vi "DAC Memory Fill [DFIL].vi"(7 "Micropulse # In":i32, 8 "error in (no error)":errorcluster, 9 "Gain (dB)":dbl min=-6.0 max=70.0 step=0.25 format="%.2fdB", 10 "End Addr":i32, 11 "Start Addr":i32) -> (0 "error out":errorcluster, 5 "Micropulse # Out":i32)   [LabVIEW 2026, in "MicroPulse_Driver.lvlib"]
doc: "Fills all addresses from address 1 to address 2 with the specified value. The addresses are within the range 0 to 65530 for standard DAC and the range 70000 to 70511 for water path DAC used in FMC echo gate mode. This command is useful for gain gating specific signals at specific ranges.\n\nParameters:\n<Addr 1> : Start address from which the specified value is to fill. Integer number between 0 and 65530 or 70000 and 70511\n\n<Addr 2> : End address to which the specified value is filled Integer number between 0 and 65530 or 70000 and 70511\n\n<Value> : Integer number representing a gain increase in 0.25 dB steps: 0 - 280 (0 - 70dB).\nThe address and value may be entered in decimal or hexadecimal Formats.\n\nExample:\nDFIL 100 200 20 : Fill from absolute address 100 to absolute address 200 with gain value 5dB.\n\nDFIL 20H C0H 120 : Fill from HEX address 20 to HEX address C0 with gain value 30.0dB"
uses:
  MicroPulse_Driver.lvlib
  Private/MP-Registry Action-Enum.ctl
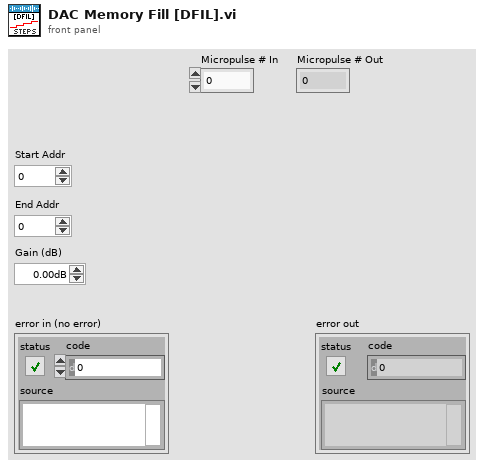
[diagram p1: front panel]
types:
  T1 = typedef "MicroPulse_Driver.lvlib/MP-Registry Action-Enum.ctl" = enum16{"Read", "Add Test", "Add Command", "Add Gate Command", "Add Encoder Command", "Clear Command  List", "Set Registry", "Set System Details", "Set DOF", "Set Velocity", "Disable Asynch Reads", "Enable Asynch Reads", "Add Connection", "Disconnect", "Shutdown"}
  T2 = typedef "MicroPulse_Driver.lvlib/TCP config.ctl" = cluster{"Connection ID":refnum<k5>, "IP address":string, "host port":u16, "OC timeout":i32, "Read timeout":i32, "Write timeout":i32}
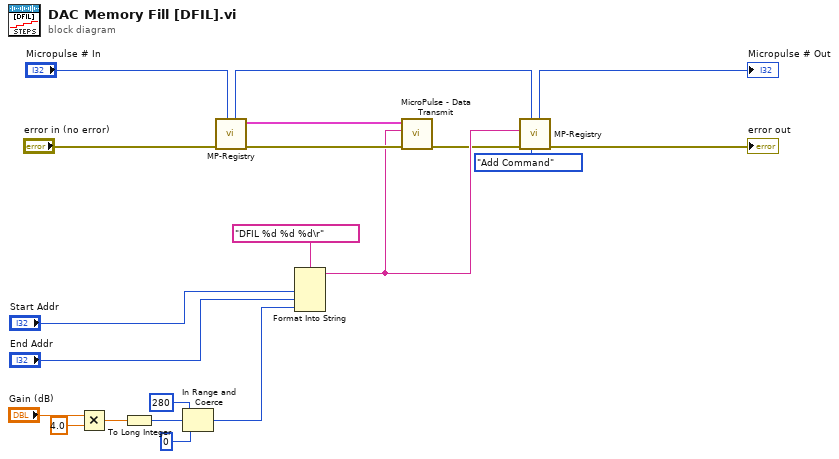
[diagram p0: block diagram]
diagram:
  n1 = Multiply(x="Gain (dB)", y=4.0) -> (x*y=w6:dbl)
  n2 = To Long Integer(number=w6) -> (32bit integer=w4:i32)
  n3 = In Range and Coerce(upper limit=280, x=w4, lower limit=0) -> (coerced(x)=w3:i32)  [unwired: 1 out]
  n4 = call "MP-Registry.vi"("Micropulse # In"="Micropulse # In", "error in (no error)"="error in (no error)") -> ("error out"=w18:errorcluster, "TCP config"=w17:T2, "Micropulse # Out"=w11:i32)  [unwired: 6 in, 1 out]
  n5 = Format Into String(format string="DFIL %d %d %d\r", "Start Addr", "End Addr", w3) -> (resulting string=w15:string)  [unwired: 2 in, 1 out]
  n6 = call "MicroPulse - Data Transmit.vi"("error in (no error)"=w18, "data"=w15, "TCP config"=w17) -> ("error out"=w13:errorcluster)  [unwired: 6 in, 2 out]
  n7 = call "MP-Registry.vi"("Action"=MP-Registry_Action-Enum."Add Command", "Micropulse # In"=w11, "error in (no error)"=w13, "Data in"=w15) -> ("error out"=→"error out":errorcluster, "Micropulse # Out"=→"Micropulse # Out":i32)  [unwired: 4 in, 2 out]
